vi "Initialize.vi"(4 "Terminal Address":T1, 6 "RT 1?":bool, 8 "error in (no error)":errorcluster, 10 "RT Commands":T2[](array[typedef]) {"Data Fields"."Base Word" format="%04d"; "Initial Data" format="%04x"}, 11 "RT Configuration":T8) -> (0 "error out":errorcluster, 3 "Remote Terminal out":refnum<class "Remote Terminal.lvclass">)   [LabVIEW 2020, in "BCI-1553 API.lvlib" / "Remote Terminal.lvclass"]
doc: "Generates a Remote Terminal object that can be used in a Component. A Component may have up one or two Remote Terminal and nothing else. If this is the first Remote Terminal on a Component, the 'RT 1?' should be set TRUE. If this is the second Remote Terminal on a Component, the 'RT 1?' parameter should be set FALSE."
uses:
  Remote Terminal.lvclass
  TypeDefs/RT Configuration.ctl
  TypeDefs/RT-RT Timeout.ctl
  TypeDefs/Mode Code 17 Sync Configuration.ctl
  TypeDefs/RT Timetag Configuration.ctl
  TypeDefs/RT Command Config.ctl
  Frames & Messages/TypeDefs/Command Type.ctl
  Frames & Messages/TypeDefs/Command SubAddress.ctl
  Frames & Messages/TypeDefs/Command Word Count.ctl
  Frames & Messages/TypeDefs/Simplified Parameter Data Table.ctl
  Frames & Messages/TypeDefs/Scaling Information.ctl
  Frames & Messages/TypeDefs/Command Terminal Address.ctl
  TypeDefs/RT CMD Config - Private.ctl
  Frames & Messages/TypeDefs/Parameter Table Data.ctl
  Remote Terminal.lvclass/Remote Terminal.ctl
  BCI-1553 API.lvlib
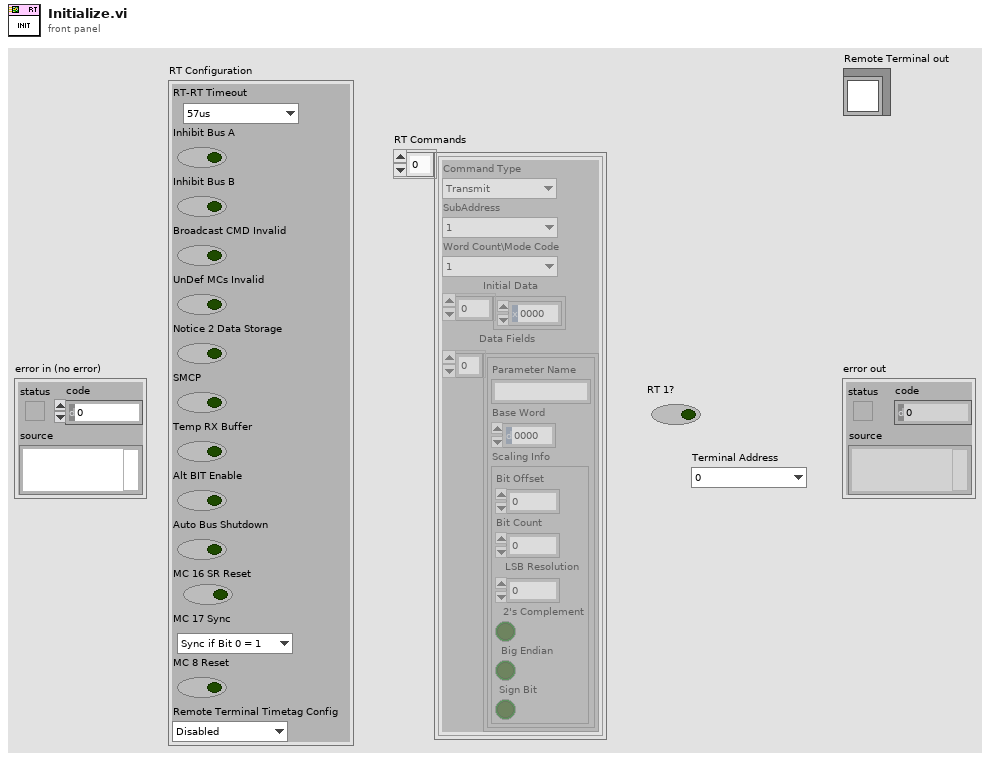
[diagram p1: front panel]
types:
  T1 = typedef "BCI-1553 API.lvlib/Command Terminal Address.ctl" = enum16{"0", "1", "2", "3", "4", "5", "6", "7", "8", "9", "10", "11", "12", "13", "14", "15", "16", "17", "18", "19", "20", "21", "22", "23", "24", "25", "26", "27", "28", "29", "30", "Broadcast"}
  T2 = typedef "BCI-1553 API.lvlib/Remote Terminal.lvclass/RT Command Config.ctl" = cluster{"Command Type":T3, "SubAddress":T4, "Word Count\\Mode Code":T5, "Initial Data":u16[], "Data Fields":T6[]}
  T3 = typedef "BCI-1553 API.lvlib/Command Type.ctl" = enum16{"Transmit", "Receive"}
  T4 = typedef "BCI-1553 API.lvlib/Command SubAddress.ctl" = enum16{"Mode Code", "1", "2", "3", "4", "5", "6", "7", "8", "9", "10", "11", "12", "13", "14", "15", "16", "17", "18", "19", "20", "21", "22", "23", "24", "25", "26", "27", "28", "29", "30"}
  T5 = typedef "BCI-1553 API.lvlib/Command Word Count.ctl" = enum16{"1", "2", "3", "4", "5", "6", "7", "8", "9", "10", "11", "12", "13", "14", "15", "16", "17", "18", "19", "20", "21", "22", "23", "24", "25", "26", "27", "28", "29", "30", "31", "32"}
  T6 = typedef "BCI-1553 API.lvlib/Simplified Parameter Data Table.ctl" = cluster{"Parameter Name":string, "Base Word":u16, "Scaling Info":T7}
  T7 = typedef "BCI-1553 API.lvlib/Scaling Information.ctl" = cluster{"Bit Offset":i32, "Bit Count":i32, "LSB Resolution":dbl, "2's Complement":bool, "Big Endian":bool, "Sign Bit":bool}
  T8 = typedef "BCI-1553 API.lvlib/Remote Terminal.lvclass/RT Configuration.ctl" = cluster{"RT-RT Timeout":T9, "Inhibit Bus A":bool, "Inhibit Bus B":bool, "Broadcast CMD Invalid":bool, "UnDef MCs Invalid":bool, "Notice 2 Data Storage":bool, "SMCP":bool, "Temp RX Buffer":bool, "Alt BIT Enable":bool, "Auto Bus Shutdown":bool, "MC 16 SR Reset":bool, "MC 17 Sync":T10, "MC 8 Reset":bool, "Remote Terminal Timetag Config":T11}
  T9 = typedef "BCI-1553 API.lvlib/Remote Terminal.lvclass/RT-RT Timeout.ctl" = enum16{"57us", "62us", "100us", "180us"}
  T10 = typedef "BCI-1553 API.lvlib/Remote Terminal.lvclass/Mode Code 17 Sync Configuration.ctl" = enum16{"Sync if Bit 0 = 1", "Sync if Bit 0 = 0", "Sync Unconditionally"}
  T11 = typedef "BCI-1553 API.lvlib/Remote Terminal.lvclass/RT Timetag Configuration.ctl" = enum16{"Disabled", "2us", "4us", "8us", "16us", "32us", "64us"}
  T12 = typedef "BCI-1553 API.lvlib/Remote Terminal.lvclass/RT CMD Config - Private.ctl" = cluster{"Command Type":T3, "SubAddress":T4, "Word Count\\Mode Code":T5, "Initial Data":u16[], "Data Fields":T13[]}
  T13 = typedef "BCI-1553 API.lvlib/Parameter Table Data.ctl" = cluster{"Parameter Name":string, "Base Word":u16, "Address":u16, "Value":u64, "Mask":u16[], "Scaling Info":T7}
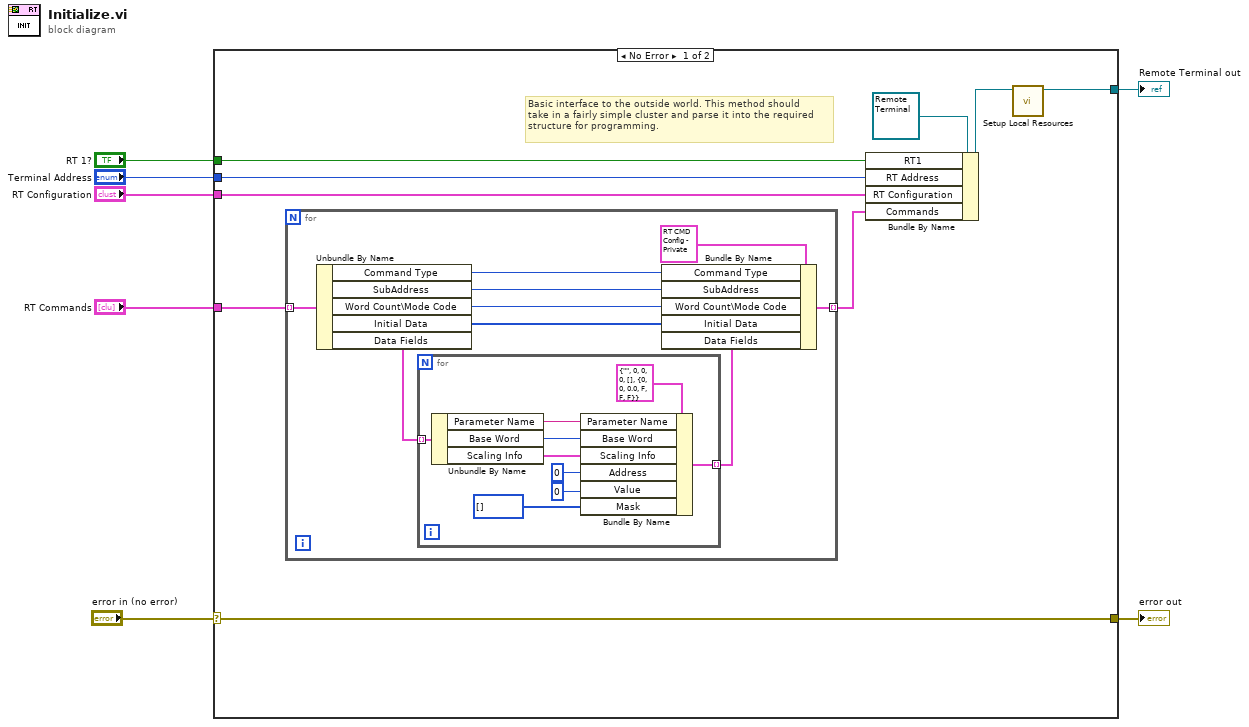
[diagram p0: block diagram]
diagram:
  n1 = case shown="No Error" "error in (no error)" {
    selector: "error in (no error)" -> [w16 w35]
    tunnel: [w16 w35] -> w6
    tunnel: [w11 _] -> w5
    tunnel: "RT 1?" -> [w15 _]
    tunnel: "Terminal Address" -> [w13 _]
    tunnel: "RT Configuration" -> [w10 _]
    tunnel: "RT Commands" -> [w9 _]
    frame No Error {
      # "Basic interface to the outside world. This method should\ntake in a fairly simple cluster and parse it into the required\nstructure for programming."
      n2 = for {
        tunnel: w9 -> [w25] mode=indexing
        tunnel: [w19] -> w8 mode=indexing
        n3 = Unbundle By Name(w25) -> ("Command Type"=w23:T3, "SubAddress"=w22:T4, "Word Count\\Mode Code"=w21:T5, "Initial Data"=w20:u16[], "Data Fields"=w18:T6[])
        n4 = for {
          tunnel: w18 -> [w32] mode=indexing
          tunnel: [w33] -> w17 mode=indexing
          n5 = Unbundle By Name(w32) -> ("Parameter Name"=w31:string, "Base Word"=w30:u16, "Scaling Info"=w26:T7)
          n6 = Bundle By Name(cluster=T13 {"Parameter Name"="", "Base Word"=0, "Address"=0, "Value"=0, "Mask"=[], "Scaling Info"={"Bit Offset"=0, "Bit Count"=0, "LSB Resolution"=0.0, "2's Complement"=FALSE, "Big Endian"=FALSE, "Sign Bit"=FALSE}} ("Parameter Table Data"), "Parameter Name"=w31, "Base Word"=w30, "Scaling Info"=w26, "Address"=u16 0, "Value"=u64 0, "Mask"=u16[] []) -> (w33:T13)
        }
        n7 = Bundle By Name(cluster=T12 {"Command Type"=enum."Transmit", "SubAddress"=enum."Mode Code", "Word Count\\Mode Code"=enum."1", "Initial Data"=[], "Data Fields"=[]} ("CMD Configuration"), "Command Type"=w23, "SubAddress"=w22, "Word Count\\Mode Code"=w21, "Initial Data"=w20, "Data Fields"=w17) -> (w19:T12)
      }
      n8 = Bundle By Name(cluster=refnum<class "Remote Terminal.lvclass"> refnum ("Remote Terminal out"), "RT1"=w15, "RT Address"=w13, "RT Configuration"=w10, "Commands"=w8) -> (w12:refnum<class "Remote Terminal.lvclass">)
      n9 = call-dynamic "Setup Local Resources.vi"("1553 SubComponent in"=w12) -> ("1553 SubComponent out"=w11:refnum<class "Remote Terminal.lvclass">)  [unwired: 9 in, 1 out]
    }
    frame Error {
    }
  }
  "error out" <- w6
  "Remote Terminal out" <- w5
